vi "Read Help Web URL.vi"(8 "error in (no error)":errorcluster, 11 "VI in":refnum<class "VI.lvclass">) -> (0 "error out":errorcluster, 2 "Help Web URL":string, 3 "VI out":refnum<class "VI.lvclass">)   [LabVIEW 2020, in "VI Properties Editor.lvlib" / "VI.lvclass"]
doc: "Gets or sets the help URL of the VI."
uses:
  VI.lvclass
  VI.lvclass/VI.ctl
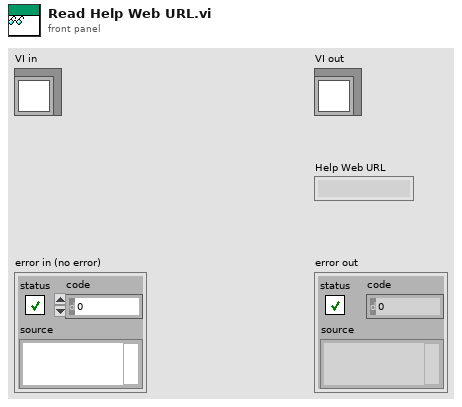
[diagram p1: front panel]
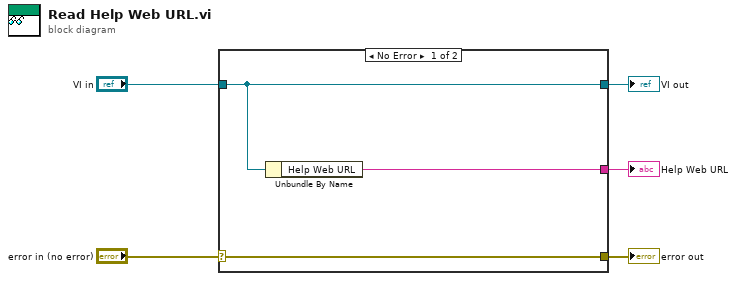
[diagram p0: block diagram]
diagram:
  n1 = case shown="No Error" "error in (no error)" {
    selector: "error in (no error)" -> [w8 w9]
    tunnel: [w8 w9] -> w4
    tunnel: [w7 w10] -> w2
    tunnel: "VI in" -> [w7 w10]
    tunnel: [w6 _] -> w1
    frame No Error {
      n2 = Unbundle By Name(w7) -> ("Help Web URL"=w6:string)
    }
    frame Error {
    }
  }
  "error out" <- w4
  "VI out" <- w2
  "Help Web URL" <- w1
